vi "Configure Alarm Com.vi"(0 "VISA resource name":refnum<visa-resource-name>, 1 "Alarm Type (0 : High limit alarm)":i32(ring) items=["High Limit Alarm (H)", "Low Limit Alarm (L)", "Delay High Limit Alarm (T)", "Delay Low Limit Alarm (t)", "Comm Los Alarm (D)"], 2 "Alarm Value (0)":i32, 3 "Enable Detect (False)":bool, 5 "Comm Channel (001)":string="001", 7 "Alarm Number (1)":i32=1 min=1 max=4 step=1, 9 "Enable Alarm (False)":bool, 11 "error in (no error)":errorcluster, 12 "Output (0 : Off)":u16(ring) items=["Off", "DO", "Internal Switch"], 13 "Relay Number (001)":string="001") -> (4 "VISA resource name out":refnum<visa-resource-name>, 6 "Comm Channel":string, 8 "Alarm Number":i32, 15 "error out":errorcluster)   [LabVIEW 2020, in "Yokogawa GX Series.lvlib"]
doc: "Sets the alarm of a communication channel.\n\nCommand: SAlarmCom"
uses:
  <instrlib>/Yokogawa GX Series/Yokogawa GX Series.lvlib
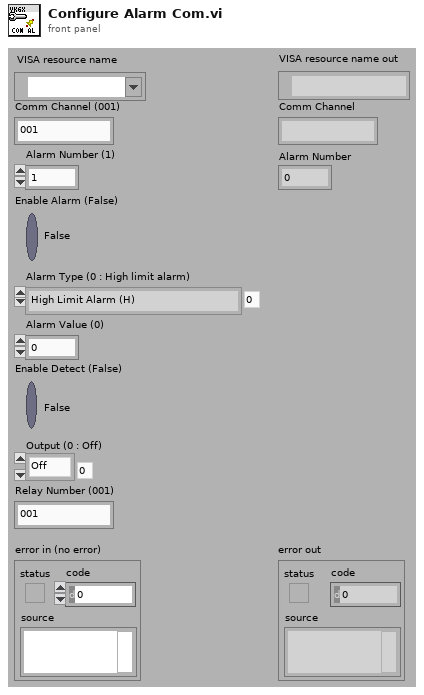
[diagram p1: front panel]
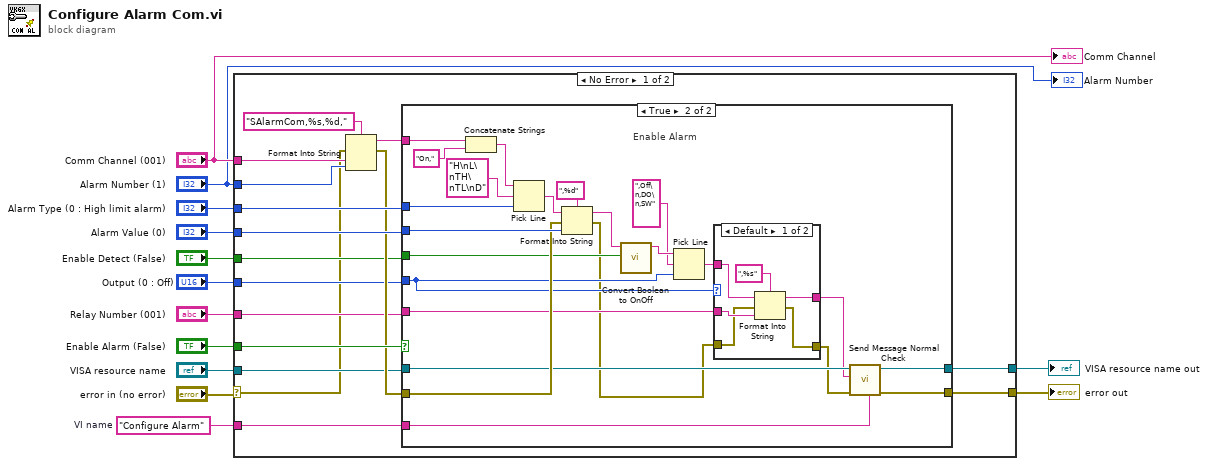
[diagram p0: block diagram]
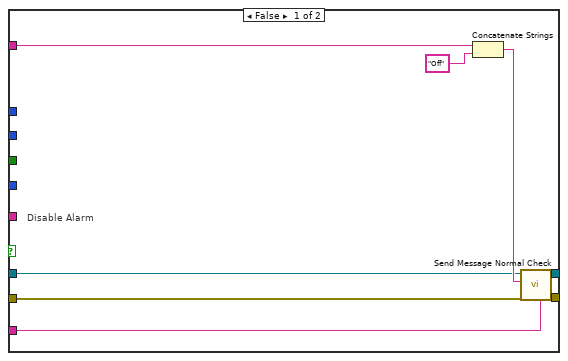
[diagram p2: hidden frame]
diagram:
  w9 = "Configure Alarm"  # VI name
  n1 = case shown="No Error" "error in (no error)" {
    selector: "error in (no error)" -> [w14 w69]
    tunnel: "Enable Alarm (False)" -> [w28 _]
    tunnel: "Alarm Type (0 : High limit alarm)" -> [w26 _]
    tunnel: "Alarm Value (0)" -> [w25 _]
    tunnel: "VISA resource name" -> [w23 w70]
    tunnel: w9 -> [w22 _]
    tunnel: [w21 w70] -> w8
    tunnel: [w20 w69] -> w7
    tunnel: "Enable Detect (False)" -> [w19 _]
    tunnel: "Relay Number (001)" -> [w18 _]
    tunnel: "Output (0 : Off)" -> [w17 _]
    tunnel: "Comm Channel (001)" -> [w16 _]
    tunnel: "Alarm Number (1)" -> [w15 _]
    frame No Error {
      n2 = Format Into String(format string="SAlarmCom,%s,%d,", error in=w14, w16, w15) -> (resulting string=w27:string, error out=w24:errorcluster)  [unwired: 1 in]
      n3 = case shown="True" w28 {
        tunnel: w27 -> [w36 w58]
        tunnel: w26 -> [_ w59]
        tunnel: w25 -> [_ w55]
        tunnel: w24 -> [w32 w54]
        tunnel: w23 -> [w34 w49]
        tunnel: w22 -> [w33 w53]
        tunnel: [w31 w47] -> w21
        tunnel: [w30 w46] -> w20
        tunnel: w19 -> [_ w48]
        tunnel: w18 -> [_ w40]
        tunnel: w17 -> [_ w43]
        frame False {
          # "Disable Alarm"
          n4 = Concatenate Strings(w36, "Off") -> (w35:string)
          n5 = call <instrlib>:"Send Message Normal Check.vi"("Source (\"\")"=w33, "error in (no error)"=w32, "Send Message (\"\")"=w35, "VISA resource name"=w34) -> ("error out"=w30:errorcluster, "VISA resource name out"=w31:refnum<visa-resource-name>)  [unwired: 2 in, 4 out]
        }
        frame True {
          # "Enable Alarm"
          n6 = Concatenate Strings(w58, "On,") -> (w51:string)
          n7 = Pick Line(string ("")=w51, multi-line string="H\nL\nTH\nTL\nD", line index=w59) -> (output string=w56:string)
          n8 = Format Into String(format string=",%d", initial string=w56, error in=w54, w55) -> (resulting string=w50:string, error out=w39:errorcluster)
          n9 = call <instrlib>:"Convert Boolean to OnOff.vi"("On/Off"=w48, "Initial String (\"\")"=w50) -> ("Resulting String"=w45:string)  [unwired: 9 in]
          n10 = Pick Line(string ("")=w45, multi-line string=",Off\n,DO\n,SW", line index=w43) -> (output string=w42:string)
          n11 = case shown="Default" w43 {
            tunnel: w42 -> [w65 w68]
            tunnel: [w62 w68] -> w41
            tunnel: w40 -> [w66 _]
            tunnel: w39 -> [w63 w67]
            tunnel: [w61 w67] -> w38
            frame Default {
              n12 = Format Into String(format string=",%s", initial string=w65, error in=w63, w66) -> (resulting string=w62:string, error out=w61:errorcluster)
            }
            frame 0 {
            }
          }
          n13 = call <instrlib>:"Send Message Normal Check.vi"("Source (\"\")"=w53, "error in (no error)"=w38, "Send Message (\"\")"=w41, "VISA resource name"=w49) -> ("error out"=w46:errorcluster, "VISA resource name out"=w47:refnum<visa-resource-name>)  [unwired: 2 in, 4 out]
        }
      }
    }
    frame Error {
    }
  }
  "error out" <- w7
  "VISA resource name out" <- w8
  "Comm Channel" <- "Comm Channel (001)"
  "Alarm Number" <- "Alarm Number (1)"
